vi "DrawBoard.vi"(9 "picture in":picture, 10 "Pieces":i32[][][](array[numeric]), 11 "Block Size":i16) -> (3 "picture out":picture)   [LabVIEW 2014]
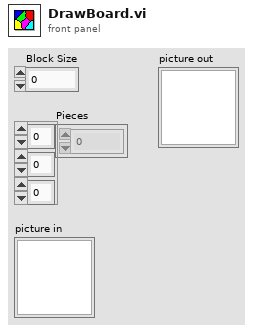
[diagram p1: front panel]
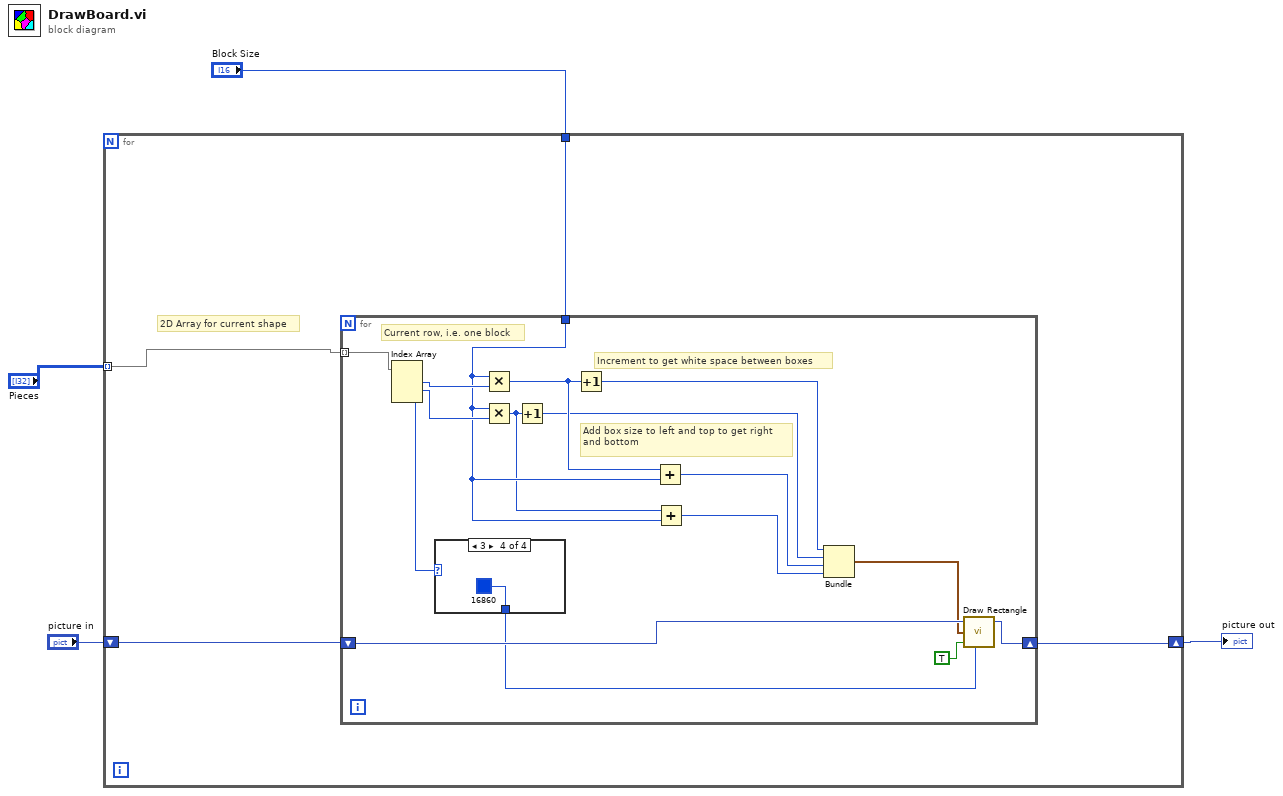
[diagram p0: block diagram]
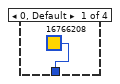
[diagram p2: hidden frame]
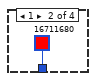
[diagram p3: hidden frame]
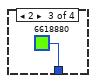
[diagram p4: hidden frame]
diagram:
  n1 = for {
    shift-right: [w5] -> w3
    shift-left: "picture in" -> [w6]
    tunnel: "Pieces" -> [w8] mode=indexing
    tunnel: "Block Size" -> [w7]
    # "2D Array for current shape"
    n2 = for {
      shift-right: [w22] -> w5
      shift-left: w6 -> [w23]
      tunnel: w8 -> [w21] mode=indexing
      tunnel: w7 -> [w17]
      # "Add box size to left and top to get right and bottom"
      # "Increment to get white space between boxes"
      # "Current row, i.e. one block"
      n3 = Index Array(array=w21) -> (element #1=w19:i32, element #2=w18:i32, element #3=w10:i32)  [unwired: 3 in]
      n4 = case shown="3" w10 {
        tunnel: [u32 16766208 u32 16711680 u32 6618880 u32 16860] -> w9
        frame 0, Default {
        }
        frame 1 {
        }
        frame 2 {
        }
        frame 3 {
        }
      }
      n5 = Multiply(x=w17, y=w19) -> (x*y=w13:i32)
      n6 = Multiply(x=w17, y=w18) -> (x*y=w12:i32)
      n7 = Increment(x=w12) -> (x+1=w11:i32)
      n8 = Increment(x=w13) -> (x+1=w16:i32)
      n9 = Add(x=w13, y=w17) -> (x+y=w15:i32)
      n10 = Add(x=w12, y=w17) -> (x+y=w14:i32)
      n11 = Bundle(w16, w11, w15, w14) -> (w20:cluster{i32, i32, i32, i32})  [unwired: 1 in]
      n12 = call <vilib>:"Draw Rectangle.vi"("picture"=w23, "rect"=w20, "fill?(F)"=TRUE, "color(black)"=w9) -> ("new picture"=w22:picture)  [unwired: 5 in]
    }
  }
  "picture out" <- w3
